vi "Sending_Other_Values_SlaveSender.vi"   [LabVIEW 2012]
uses:
  <vilib>/NXT/Block Support/HWPage.SensorType.ctl
  <vilib>/NXT/Block Support/HWPage.SensorMode.ctl
  <vilib>/NXT/Block Support/NXT_InputPort.ctl
  <vilib>/NXT/Subs/MotorOutput.ctl
  <vilib>/NXT/Dual Mode Library/Sensors/i2c_sensors_big.vi
types:
  T1 = typedef "NXT_InputPort.ctl" = u8
  T2 = typedef "HWPage.SensorType.ctl" = u8
  T3 = typedef "HWPage.SensorMode.ctl" = u8
  T4 = typedef "LVHSConnector.ctl" = cluster{"Hardware":string, "Flattened String":string}
  T5 = typedef "MotorOutput.ctl" = u8
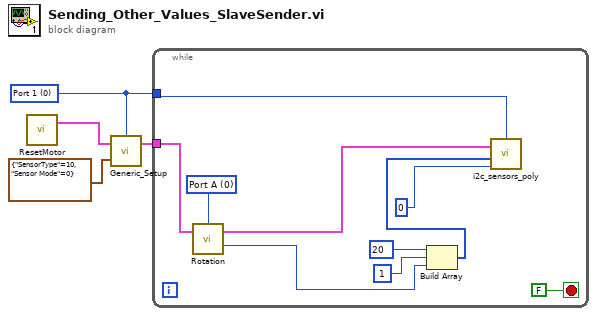
[diagram p0: block diagram]
diagram:
  w2 = T1 0 items=["Port 1", "Port 2", "Port 3", "Port 4"] ("Port")
  n1 = call <vilib>:"ResetMotor.vi"() -> ("NXT"=w1:T4)  [unwired: 4 in]
  n2 = call <vilib>:"Generic_Setup.vi"("Sensor Setup"=cluster{"SensorType":T2, "Sensor Mode":T3} {"SensorType"=10, "Sensor Mode"=0}, "NXT"=w1, "Port"=w2) -> ("NXT"=w3:T4)  [unwired: 1 out]
  n3 = while {
    tunnel: w3 -> [w7]
    tunnel: w2 -> [w13]
    stop <- FALSE stop-if-true
    w8 = T5 0 items=["Port A"=0, "Port B"=1, "Port C"=2, "Ports A & B"=4, "Ports A & C"=5, "Ports B & C"=6, "All Ports"=3] ("Output Port (All Ports)")
    n4 = call <vilib>:"Rotation.vi"("NXT"=w7, "Port (Port A)"=w8) -> ("Angle of Rotation"=w5:i32, "NXT"=w6:T4)  [unwired: 1 in]
    n5 = Build Array(u8 20, 1, w5) -> (w9:i32[])
    n6 = call-poly <vilib>:"i2c_sensors_poly.vi"("Return Length"=u8 0, "Bytes to Write"=w9, "NXT"=w6, "Port"=w13) -> ()  [unwired: 1 in, 3 out]
  }
